vi "Flatten XML String.vi"(7 "Root ID":string, 8 "Error In":errorcluster, 11 "Tree":refnum<data-value>) -> (0 "Error Out":errorcluster, 1 "XML String":string, 3 "Tree":refnum<data-value>)   [LabVIEW 2017, in "Tree API.lvlib" / "Tree.lvclass"]
doc: "Flatten the specified Tree to XML representation. Any existing Tree can be used as the Root element in XML representation. This method can be used to copy contents of one Tree Manager to another.\n\n<b>WARNING</b> This methods implements basic LV implementaion for parsing the XML. It is supported on multiple targets because it does not use the native LV DOM parser. This means it might be less optimal and not handle all XML parsing errors. Please test it extensively before using in your final design.\n\n<b>WARNING</b> All Tree names that contain a space character will have it replaced by underscore character. This is required by XML specification."
uses:
  Tree.lvclass
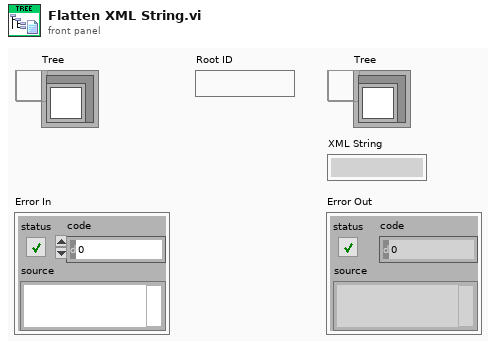
[diagram p1: front panel]
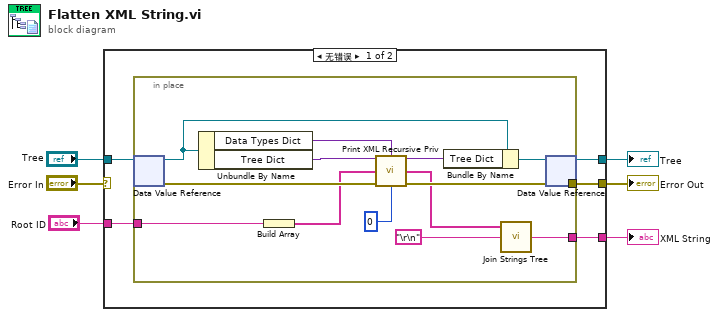
[diagram p0: block diagram]
diagram:
  n1 = case shown="无错误" "Error In" {
    selector: "Error In" -> [_ w25]
    tunnel: "Tree" -> [w11 w26]
    tunnel: [w10 w26] -> w5
    tunnel: [w9 w25] -> w3
    tunnel: "Root ID" -> [w8 _]
    tunnel: [w7 _] -> w1
    frame No Error {
      n2 = in-place {
        in-place-border: [w23] -> w9
        in-place-border: w8 -> [w20]
        in-place-border: [w12] -> w7
        n3 = in-place-dvr #1(w11) -> (w24:refnum<class "Tree.lvclass">, w21:errorcluster)
        n4 = Unbundle By Name(w24) -> ("Data Types Dict"=w16:variant, "Tree Dict"=w19:variant)
        n5 = Build Array(w20) -> (w17:string[])
        n6 = call "Print XML Recursive Priv.vi"("Tree Dictionary In"=w19, "Data Types Dict"=w16, "Child IDs"=w17, "error in"=w21, "Indent"=0) -> ("Tree Dictionary Out"=w18:variant, "XML Lines"=w13:string[], "error out"=w23:errorcluster)  [unwired: 8 in]
        n7 = Bundle By Name(cluster=w24, "Tree Dict"=w18) -> (w22:refnum<class "Tree.lvclass">)
        n8 = call "Join Strings Tree.vi"("Separator (,)"="\r\n", "Strings In"=w13) -> ("String"=w12:string)  [unwired: 1 in]
        n9 = in-place-dvr #1(w22) -> (w10:refnum<data-value>)  [unwired: 1 out]
      }
    }
    frame Error {
    }
  }
  "Tree" <- w5
  "Error Out" <- w3
  "XML String" <- w1
